vi "Create.vi"(8 "error in (no error)":errorcluster) -> (0 "error out":errorcluster, 2 "Event Registration Refnum":refnum<event-registration>, 3 "Status Updater out":refnum<class "Status Updater.lvclass">)   [LabVIEW 2014, in "Status Updater.lvclass"]
uses:
  Status Updater.lvclass
  Status Updater.lvclass/Status Updater.ctl
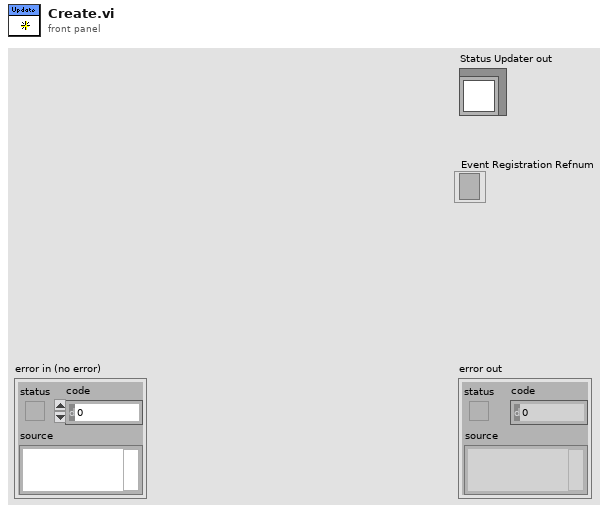
[diagram p1: front panel]
types:
  T1 = cluster{"Build Text":refnum<user-event>, "Progress":refnum<user-event>}
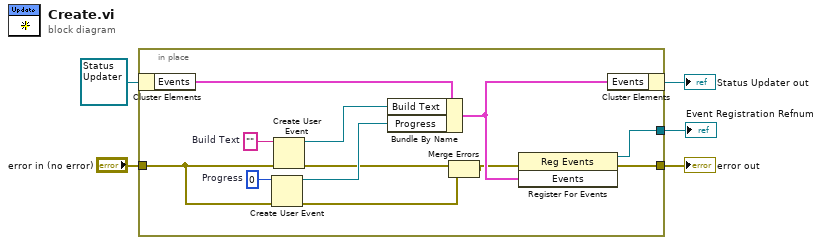
[diagram p0: block diagram]
diagram:
  n1 = in-place {
    in-place-border: "error in (no error)" -> [w9]
    in-place-border: [w8] -> w2
    in-place-border: [w6] -> w1
    w15 = u32 0  # Progress
    w17 = ""  # Build Text
    n2 = in-place-cluster #1(refnum<class "Status Updater.lvclass"> refnum ("Status Updater in")) -> ("Events"=w13:T1)
    n3 = Create User Event(user event datatype=w15, error in=w9) -> (user event=w14:refnum<user-event>, error out=w10:errorcluster)
    n4 = Create User Event(user event datatype=w17, error in=w9) -> (user event=w16:refnum<user-event>, error out=w11:errorcluster)
    n5 = Bundle By Name(cluster=w13, "Build Text"=w16, "Progress"=w14) -> (w12:T1)
    n6 = Merge Errors(w11, w10) -> (w7:errorcluster)
    n7 = register-events(error in=w7, w12) -> (reference out=w6:refnum<event-registration>, error out=w8:errorcluster)  [unwired: 1 in]
    n8 = in-place-cluster #1("Events"=w12) -> (→"Status Updater out":refnum<class "Status Updater.lvclass">)
  }
  "error out" <- w2
  "Event Registration Refnum" <- w1
